vi "IN_6517B.vi"(1 "Ctl Refnum 2":refnum<vi>, 2 "Ctl Refnum":refnum<vi>, 7 "Cluster":T2, 8 "error in (no error)":errorcluster caption="错误输入（无错误）", 9 "Temp. Adr.":refnum<visa-resource-name> caption="温度计地址", 10 "6517 Adr.":refnum<visa-resource-name> caption="6517地址", 11 "引用句柄输出":refnum<file>) -> (6 "Cluster 2":T1)   [LabVIEW 2017]
panel:
  out "Temperture-Time":cluster{dbl[], dbl[]}(graph)
  out "Present Current (A)":dbl
  out "Time (s)":dbl
  out "Resistivity (ohm·cm)":dbl
  out "电阻 (ohm)":dbl
  in  "电压(V)":dbl
  out "当前温度(°C)":dbl=311.11
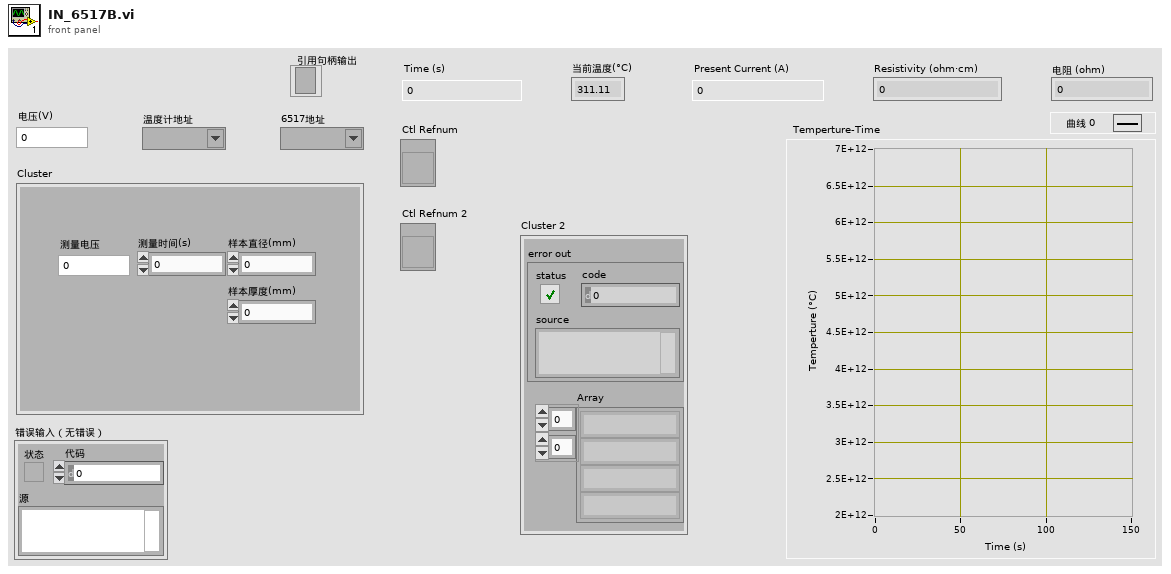
[diagram p1: front panel]
types:
  T1 = cluster{"Array":string[][], "error out":errorcluster}
  T2 = cluster{"测量时间(s)":dbl, "测量电压":dbl, "样本直径(mm)":dbl, "样本厚度(mm)":dbl}
  T3 = cluster{dbl, "PV":dbl, "Resistance (ohm)":dbl, dbl}
  T4 = cluster{"Array 2":string[][], "error out":errorcluster}
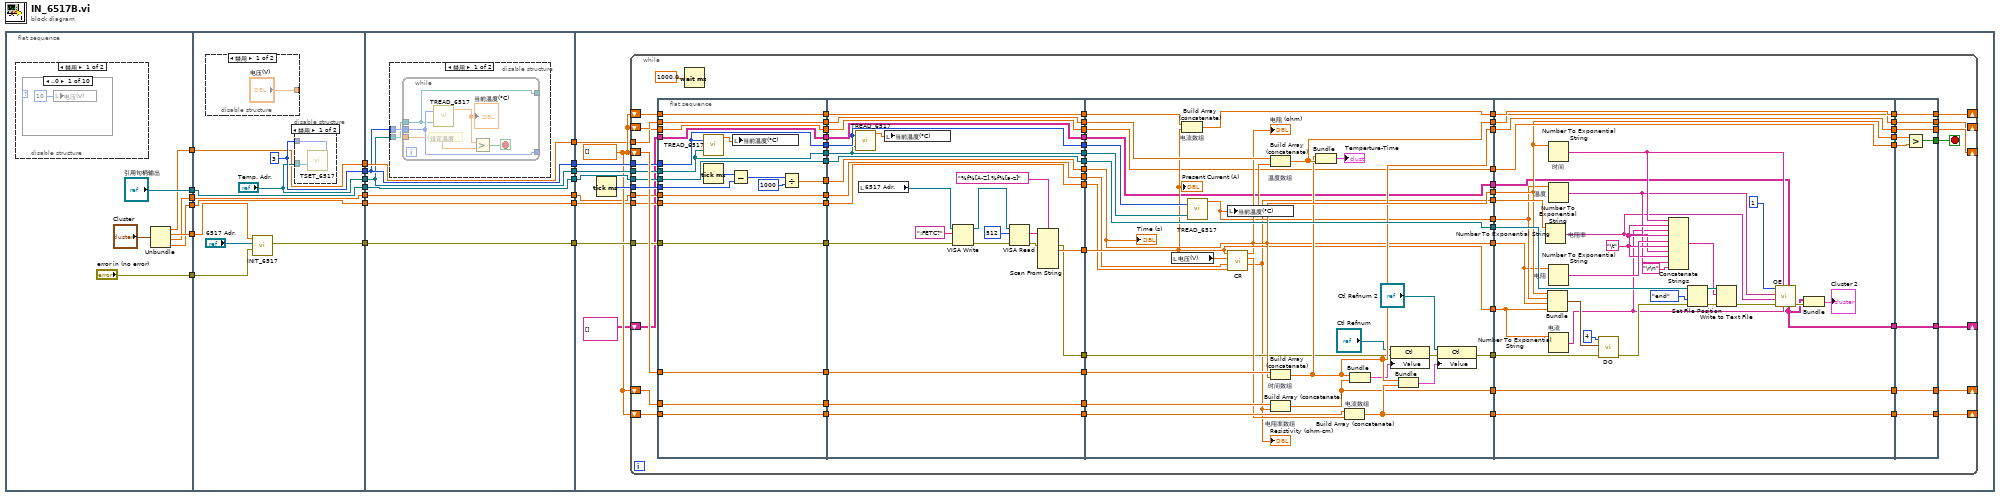
[diagram p0: block diagram]
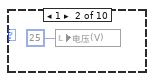
[diagram p2: hidden frame]
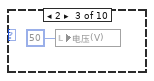
[diagram p3: hidden frame]
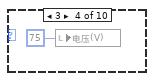
[diagram p4: hidden frame]
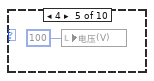
[diagram p5: hidden frame]
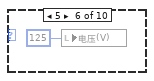
[diagram p6: hidden frame]
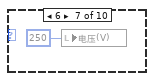
[diagram p7: hidden frame]
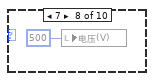
[diagram p8: hidden frame]
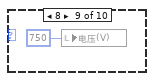
[diagram p9: hidden frame]
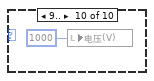
[diagram p10: hidden frame]
diagram:
  n1 = flat-sequence {
    tunnel: ["引用句柄输出"] -> w20
    tunnel: ["error in (no error)"] -> w12
    tunnel: [w24] -> w9
    tunnel: [w22] -> w5
    tunnel: [w21] -> w3
    tunnel: [w23] -> w2
    tunnel: w20 -> [w45]
    tunnel: [w45] -> w19
    tunnel: [w43] -> w18
    tunnel: ["Temp. Adr."] -> w17
    tunnel: [w47] -> w16
    tunnel: w12 -> [w44]
    tunnel: [w41] -> w10
    tunnel: w9 -> [w41]
    tunnel: [w40] -> w6
    tunnel: w5 -> [w40]
    tunnel: [w39] -> w4
    tunnel: w3 -> [w39]
    tunnel: w2 -> [w38]
    tunnel: w19 -> [w57]
    tunnel: w18 -> [w56]
    tunnel: w17 -> [w51]
    tunnel: w16 -> [w52]
    tunnel: [w57] -> w15
    tunnel: [w56] -> w14
    tunnel: [w51] -> w13
    tunnel: [w55] -> w11
    tunnel: w10 -> [w55]
    tunnel: [w54] -> w8
    tunnel: [w53] -> w7
    tunnel: w6 -> [w54]
    tunnel: w4 -> [w53]
    tunnel: [w52] -> w1
    tunnel: w15 -> [w73]
    tunnel: w14 -> [w72]
    tunnel: w13 -> [w70]
    tunnel: w11 -> [w68]
    tunnel: w8 -> [w67]
    tunnel: w7 -> [w66]
    tunnel: w1 -> [w71]
    frame #0 {
      n2 = disable-structure shown="禁用" {
        frame Disabled {
          n3 = case shown="..0" {
            selector: _ -> [_ _ _ _ _ _ _ _ _ _]
            frame ..0 {
              n4 = local write "电压(V)"(10) -> ()
            }
            frame 1 {
              n5 = local write "电压(V)"(25) -> ()
            }
            frame 2 {
              n6 = local write "电压(V)"(50) -> ()
            }
            frame 3 {
              n7 = local write "电压(V)"(75) -> ()
            }
            frame 4 {
              n8 = local write "电压(V)"(100) -> ()
            }
            frame 5 {
              n9 = local write "电压(V)"(125) -> ()
            }
            frame 6 {
              n10 = local write "电压(V)"(250) -> ()
            }
            frame 7 {
              n11 = local write "电压(V)"(500) -> ()
            }
            frame 8 {
              n12 = local write "电压(V)"(750) -> ()
            }
            frame 9.. {
              n13 = local write "电压(V)"(1000) -> ()
            }
          }
        }
        frame Enabled {
        }
      }
      n14 = Unbundle("Cluster") -> ("测量时间(s)"=w24:dbl, "测量电压"=w23:dbl, "样本直径(mm)"=w22:dbl, "样本厚度(mm)"=w21:dbl)
    }
    frame #1 {
      w47 = i8 3 ("Address No.")
      n15 = disable-structure shown="禁用" {
        disable-tunnel: ["电压(V)" _] -> _
        frame Disabled {
        }
        frame Enabled {
        }
      }
      n16 = call "INIT_6517.vi"("error in (no error)"=w44, "VISA resource name"="6517 Adr.", "Vin"=w38) -> ("error out"=w43:errorcluster)  [unwired: 7 in, 1 out]
      n17 = disable-structure shown="禁用" {
        disable-tunnel: w47 -> [w49 _]
        disable-tunnel: "Temp. Adr." -> [w48 _]
        frame Disabled {
          n18 = call "TSET_6517.vi"("Address No."=w49, "VISA resource name"=w48) -> ()  [unwired: 10 in]
        }
        frame Enabled {
        }
      }
    }
    frame #2 {
      n19 = disable-structure shown="禁用" {
        disable-tunnel: w52 -> [w59 _]
        disable-tunnel: w51 -> [w58 _]
        frame Disabled {
          n20 = while {
            tunnel: w58 -> [w61]
            tunnel: w59 -> [w62]
            tunnel: [w62] -> _
            tunnel: [w61] -> _
            tunnel: _ -> [w60]
            stop <- w63 stop-if-true
            # "设定温度"
            n21 = call "TREAD_6517.vi"("Address No."=w62, "VISA resource name"=w61) -> ("PV"=w64:dbl)  [unwired: 3 out]
            "当前温度(°C)" <- w64
            n22 = Greater?(x=w64, y=w60) -> (0:w63:bool)
          }
        }
        frame Enabled {
        }
      }
    }
    frame #3 {
      w69 = dbl[] []
      n23 = Tick Count (ms)() -> (millisecond timer value=w74:u32)
      n24 = while {
        tunnel: w74 -> [w147]
        shift-right: [w145] -> _
        shift-left: w69 -> [w146]
        shift-right: [w140] -> _
        shift-left: w69 -> [w144]
        shift-right: [w143] -> _
        shift-left: w69 -> [w142]
        tunnel: w73 -> [w139]
        tunnel: w72 -> [w138]
        tunnel: w71 -> [w137]
        tunnel: w70 -> [w136]
        shift-right: [w134] -> _
        shift-left: w69 -> [w135]
        shift-right: [w98] -> _
        shift-left: w69 -> [w95]
        tunnel: w68 -> [w88]
        tunnel: w67 -> [w83]
        tunnel: w66 -> [w82]
        shift-right: [w80] -> _
        shift-left: string[][] [] -> [w75]
        stop <- w141 stop-if-true
        n25 = flat-sequence {
          tunnel: w147 -> [w165]
          tunnel: w138 -> [w152]
          tunnel: w146 -> [w159]
          tunnel: w144 -> [w158]
          tunnel: w142 -> [w157]
          tunnel: w139 -> [w156]
          tunnel: w137 -> [w161]
          tunnel: w136 -> [w160]
          tunnel: w135 -> [w155]
          tunnel: [w152] -> w133
          tunnel: [w159] -> w132
          tunnel: [w158] -> w131
          tunnel: [w157] -> w130
          tunnel: [w156] -> w129
          tunnel: [w162] -> w128
          tunnel: [w155] -> w127
          tunnel: [w161] -> w126
          tunnel: [w160] -> w125
          tunnel: [w154] -> w96
          tunnel: w95 -> [w154]
          tunnel: [w151] -> w89
          tunnel: w88 -> [w151]
          tunnel: [w150] -> w85
          tunnel: [w149] -> w84
          tunnel: w83 -> [w150]
          tunnel: w82 -> [w149]
          tunnel: [w148] -> w76
          tunnel: w75 -> [w148]
          tunnel: w133 -> [w171]
          tunnel: w132 -> [w179]
          tunnel: w131 -> [w178]
          tunnel: w130 -> [w177]
          tunnel: w129 -> [w176]
          tunnel: w128 -> [w175]
          tunnel: w127 -> [w174]
          tunnel: w126 -> [w181]
          tunnel: w125 -> [w180]
          tunnel: [w179] -> w124
          tunnel: [w178] -> w123
          tunnel: [w177] -> w122
          tunnel: [w176] -> w121
          tunnel: [w175] -> w120
          tunnel: [w184] -> w119
          tunnel: [w182] -> w118
          tunnel: [w174] -> w117
          tunnel: [w181] -> w116
          tunnel: [w180] -> w115
          tunnel: [w173] -> w99
          tunnel: w96 -> [w173]
          tunnel: [w170] -> w90
          tunnel: w89 -> [w170]
          tunnel: [w169] -> w87
          tunnel: [w168] -> w86
          tunnel: w85 -> [w169]
          tunnel: w84 -> [w168]
          tunnel: [w167] -> w77
          tunnel: w76 -> [w167]
          tunnel: w124 -> [w223]
          tunnel: w123 -> [w222]
          tunnel: w122 -> [w221]
          tunnel: w121 -> [w213]
          tunnel: w120 -> [w219]
          tunnel: w119 -> [w209]
          tunnel: w118 -> [w196]
          tunnel: w117 -> [w218]
          tunnel: w116 -> [w216]
          tunnel: w115 -> [w215]
          tunnel: [w211] -> w114
          tunnel: [w205] -> w113
          tunnel: [w220] -> w112
          tunnel: [w213] -> w111
          tunnel: [w219] -> w110
          tunnel: [w193] -> w109
          tunnel: [w209] -> w108
          tunnel: [w197] -> w107
          tunnel: [w214] -> w106
          tunnel: [w210] -> w100
          tunnel: w99 -> [w212]
          tunnel: [w206] -> w94
          tunnel: [w204] -> w93
          tunnel: [w203] -> w91
          tunnel: w90 -> [w203]
          tunnel: w87 -> [w202]
          tunnel: w86 -> [w201]
          tunnel: [w192] -> w78
          tunnel: w77 -> [w192]
          tunnel: w114 -> [w250]
          tunnel: w113 -> [w249]
          tunnel: w112 -> [w248]
          tunnel: w111 -> [w256]
          tunnel: w110 -> [w241]
          tunnel: w109 -> [w251]
          tunnel: w108 -> [w238]
          tunnel: w107 -> [w235]
          tunnel: w106 -> [w247]
          tunnel: [w250] -> w105
          tunnel: [w249] -> w104
          tunnel: [w248] -> w103
          tunnel: [w241] -> w102
          tunnel: [w247] -> w101
          tunnel: w100 -> [w246]
          tunnel: [w246] -> w97
          tunnel: w94 -> [w239]
          tunnel: w93 -> [w240]
          tunnel: [w242] -> w92
          tunnel: w91 -> [w242]
          tunnel: [w225] -> w79
          tunnel: w78 -> [w227]
          tunnel: [w263] -> w145
          tunnel: [w262] -> w140
          tunnel: [w261] -> w143
          tunnel: [w264] -> w141
          tunnel: [w260] -> w134
          tunnel: w105 -> [w263]
          tunnel: w104 -> [w262]
          tunnel: w103 -> [w261]
          tunnel: w102 -> [w265]
          tunnel: w101 -> [w260]
          tunnel: [w259] -> w98
          tunnel: w97 -> [w259]
          tunnel: w92 -> [w258]
          tunnel: [w257] -> w80
          tunnel: w79 -> [w257]
          frame #0 {
            n26 = call "TREAD_6517.vi"("Address No."=w161, "VISA resource name"=w160) -> ("PV"=w153:dbl)  [unwired: 3 out]
            n27 = Tick Count (ms)() -> (millisecond timer value=w166:u32)
            n28 = Subtract(x=w166, y=w165) -> (x-y=w164:u32)
            n29 = local write "当前温度(°C)"(w153) -> ()
            n30 = Divide(x=w164, y=u32 1000) -> (x/y=w162:dbl)
          }
          frame #1 {
            n31 = call "TREAD_6517.vi"("Address No."=w181, "VISA resource name"=w180) -> ("PV"=w172:dbl)  [unwired: 3 out]
            n32 = local read "6517 Adr."() -> (w191:refnum<visa-resource-name>)
            n33 = local write "当前温度(°C)"(w172) -> ()
            n34 = VISA Write(VISA resource name=w191, write buffer=":FETC?" ("写入缓冲区"), error in (no error)=w171) -> (VISA resource name out=w188:refnum<visa-resource-name>, error out=w189:errorcluster)  [unwired: 1 out]
            n35 = VISA Read(VISA resource name=w188, byte count=u32 512 ("字节总数"), error in (no error)=w189) -> (read buffer=w186:string, error out=w183:errorcluster)  [unwired: 2 out]
            n36 = Scan From String(format string="%f%[A-Z],%f%[a-z]" ("格式字符串"), input string=w186, error in=w183) -> (error out=w182:errorcluster, output 1=w184:dbl)  [unwired: 1 in, 9 out]
          }
          frame #2 {
            n37 = local read "电压(V)"() -> (w208:dbl)
            n38 = Build Array (concatenate) "电流数组"(w221, w209) -> (w220:dbl[])
            n39 = call "TREAD_6517.vi"("Address No."=w216, "VISA resource name"=w215) -> ("PV"=w204:dbl)  [unwired: 3 out]
            n40 = local write "当前温度(°C)"(w204) -> ()
            n41 = call "CR.vi"("Sample Thickness (mm)"=w201, "Sample Diameter (mm)"=w202, "电压(V)"=w208, "电流(A)"=w209) -> ("Resistivity (ohm·cm)"=w193:dbl, "Current (A)"=w207:dbl, "Resistance (ohm)"=w206:dbl)  [unwired: 5 in]
            "Resistivity (ohm·cm)" <- w193
            "电阻 (ohm)" <- w206
            n42 = Build Array (concatenate) "温度数组"(w218, w204) -> (w214:dbl[])
            n43 = Build Array (concatenate) "时间数组"(w223, w219) -> (w211:dbl[])
            n44 = Build Array (concatenate) "电阻率数组"(w222, w193) -> (w205:dbl[])
            n45 = Bundle(w211, w214) -> (→"Temperture-Time":cluster{dbl[], dbl[]})  [unwired: 1 out]
            n46 = Build Array (concatenate) "电流数组"(w212, w207) -> (w210:dbl[])
            n47 = Bundle(w211, w205) -> (w194:cluster{dbl[], dbl[]})  [unwired: 1 out]
            n48 = property class="Ctl"(reference="Ctl Refnum", error in=w196, "Value"=w194) -> (error out=w198:errorcluster)  [unwired: 1 out]
            n49 = Bundle(w211, w210) -> (w195:cluster{dbl[], dbl[]})  [unwired: 1 out]
            n50 = property class="Ctl"(reference="Ctl Refnum 2", error in=w198, "Value"=w195) -> (error out=w197:errorcluster)  [unwired: 1 out]
            "Present Current (A)" <- w209
            "Time (s)" <- w219
          }
          frame #3 {
            w243 = "\t"
            n51 = Number To Exponential String "电阻率"(number=w251) -> (E-format string=w230:string)  [unwired: 3 out]
            n52 = Bundle(w241, "PV"=w240, "Resistance (ohm)"=w239, w238) -> (w237:T3)  [unwired: 1 in]
            n53 = Number To Exponential String "时间"(number=w241) -> (E-format string=w232:string)  [unwired: 1 in, 2 out]
            n54 = Number To Exponential String "温度"(number=w240) -> (E-format string=w231:string)  [unwired: 3 out]
            n55 = Number To Exponential String "电阻"(number=w239) -> (E-format string=w245:string)  [unwired: 1 in, 2 out]
            n56 = Number To Exponential String "电流"(number=w238) -> (E-format string=w228:string)  [unwired: 3 out]
            n57 = call "DO.vi"("error in (no error)"=w235, "数据输出"=w237, "功能编号"=4) -> ("error out"=w234:errorcluster)  [unwired: 8 in]
            n58 = Concatenate Strings(w232, w243, w228, w243, w245, w243, w230, w243, w231, "\r\n") -> (w253:string)
            n59 = Set File Position(refnum=w256, from (0:start)=enum16{"start", "end", "current"}."end" ("自（0:起始）"), error in=w234) -> (refnum out=w254:refnum<file>, error out=w252:errorcluster)  [unwired: 1 out]
            n60 = Write to Text File(file (use dialog)=w254, text=w253, error in=w252) -> (error out=w229:errorcluster)  [unwired: 1 in, 2 out]
            n61 = call "OE.vi"("Array"=w227, "String 4"=w228, "String"=w232, "error in (no error)"=w229, "String 3"=w230, "String 2"=w231, "Numeric"=1) -> ("error out"=w226:errorcluster, "Array 2"=w225:string[][])  [unwired: 2 in, 1 out]
            n62 = Bundle("Array 2"=w225, "error out"=w226) -> (→"Cluster 2":T4)  [unwired: 1 in]
          }
          frame #4 {
            n63 = Greater?(x=w265, y=w258) -> (0:w264:bool)
          }
        }
        n64 = Wait (ms)(milliseconds to wait=1000.0 ("y")) -> ()  [unwired: 1 out]
      }
    }
  }
